vi "Get IDs.vi"(8 "error in (no error)":errorcluster, 11 "Tool Data in":refnum<class "Tool Data.lvclass">) -> (0 "error out":errorcluster, 2 "IDs":T1, 3 "Tool Data out":refnum<class "Tool Data.lvclass">)   [LabVIEW 2019, in "Tool Data.lvclass"]
uses:
  Tool Data.lvclass
  Parse/Rectangle/Rectangle.lvclass
  Parse/ParsePaths/Path.lvclass
  Parse/Dot/Dot.lvclass
  Parse/Image/SVGImage.lvclass
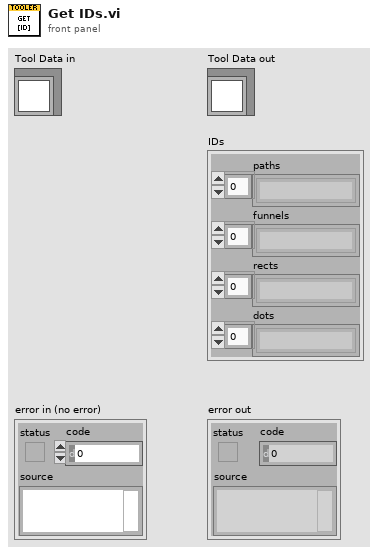
[diagram p1: front panel]
types:
  T1 = cluster{"paths":string[], "funnels":string[], "rects":string[], "dots":string[]}
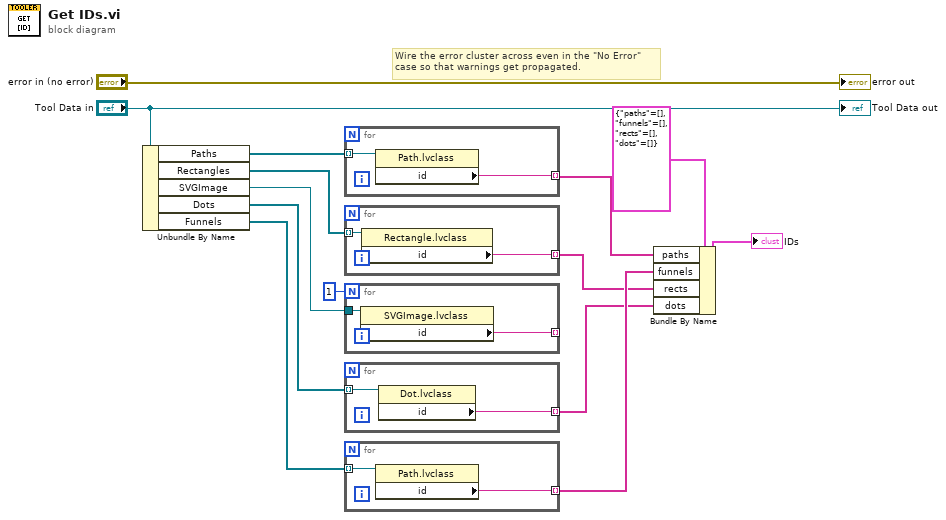
[diagram p0: block diagram]
diagram:
  # "Wire the error cluster across even in the \"No Error\"\ncase so that warnings get propagated."
  n1 = Unbundle By Name("Tool Data in") -> ("Paths"=w12:refnum<class "Path.lvclass">[], "Rectangles"=w11:refnum<class "Rectangle.lvclass">[], "SVGImage"=w10:refnum<class "SVGImage.lvclass">, "Dots"=w9:refnum<class "Dot.lvclass">[], "Funnels"=w8:refnum<class "Path.lvclass">[])
  n2 = for {
    tunnel: w12 -> [w16] mode=indexing
    tunnel: [w15] -> w5 mode=indexing
    n3 = property class="Path.lvclass"(reference=w16) -> ("id"=w15:string)  [unwired: 1 in, 2 out]
  }
  n4 = for {
    tunnel: w11 -> [w18] mode=indexing
    tunnel: [w17] -> _ mode=indexing
    tunnel: [w17] -> w2 mode=indexing
    n5 = property class="Rectangle.lvclass"(reference=w18) -> ("id"=w17:string)  [unwired: 1 in, 2 out]
  }
  n6 = for {
    N: 1 -> [_]
    tunnel: w10 -> [w20]
    tunnel: [w19] -> _ mode=indexing
    n7 = property class="SVGImage.lvclass"(reference=w20) -> ("id"=w19:string)  [unwired: 1 in, 2 out]
  }
  n8 = for {
    tunnel: w9 -> [w22] mode=indexing
    tunnel: [w21] -> w3 mode=indexing
    n9 = property class="Dot.lvclass"(reference=w22) -> ("id"=w21:string)  [unwired: 1 in, 2 out]
  }
  n10 = for {
    tunnel: w8 -> [w24] mode=indexing
    tunnel: [w23] -> w4 mode=indexing
    n11 = property class="Path.lvclass"(reference=w24) -> ("id"=w23:string)  [unwired: 1 in, 2 out]
  }
  n12 = Bundle By Name(cluster=T1 {"paths"=[], "funnels"=[], "rects"=[], "dots"=[]} ("IDs"), "paths"=w5, "funnels"=w4, "rects"=w2, "dots"=w3) -> (→"IDs":T1)
  "error out" <- "error in (no error)"
  "Tool Data out" <- "Tool Data in"
